vi "Measure_FUN_VISA.vi"(7 "VISA Action":T2, 8 "Error In":errorcluster, 10 "VISA Paremeter":T3={"Baud rate"=19200, "Data bits"=8, "Parity"=enum."None", "Stop bits"=10, "Flow control"=0} {"Flow control" items=["None"=0, "XON/XOFF"=1, "RTS/CTS"=2, "DTR/DSR"=4]; "Stop bits" items=["1.0"=10, "1.5"=15, "2.0"=20]; "Data bits" min=5 max=8 step=1; "Baud rate" items=["75"=75, "110"=110, "134"=134, "150"=150, "300"=300, "600"=600, "1200"=1200, "1800"=1800, "2400"=2400, "4800"=4800, "7200"=7200, "9600"=9600, "14400"=14400, "19200"=19200, "28800"=28800, "38400"=38400, "56000"=56000, "57600"=57600, "115200"=115200, "128000"=128000, "230400"=230400]}, 11 "VISA In":refnum<visa-resource-name>="COM9") -> (0 "Error Out":errorcluster, 2 "State":T1, 3 "VISA Out":refnum<visa-resource-name>="COM9")   [LabVIEW 2015]
uses:
  Control_Measure_VISA action.ctl
  <vilib>/Instr/_visa.llb/VISA Configure Serial Port (Instr).vi
panel:
  in  "Time out":u32=3000
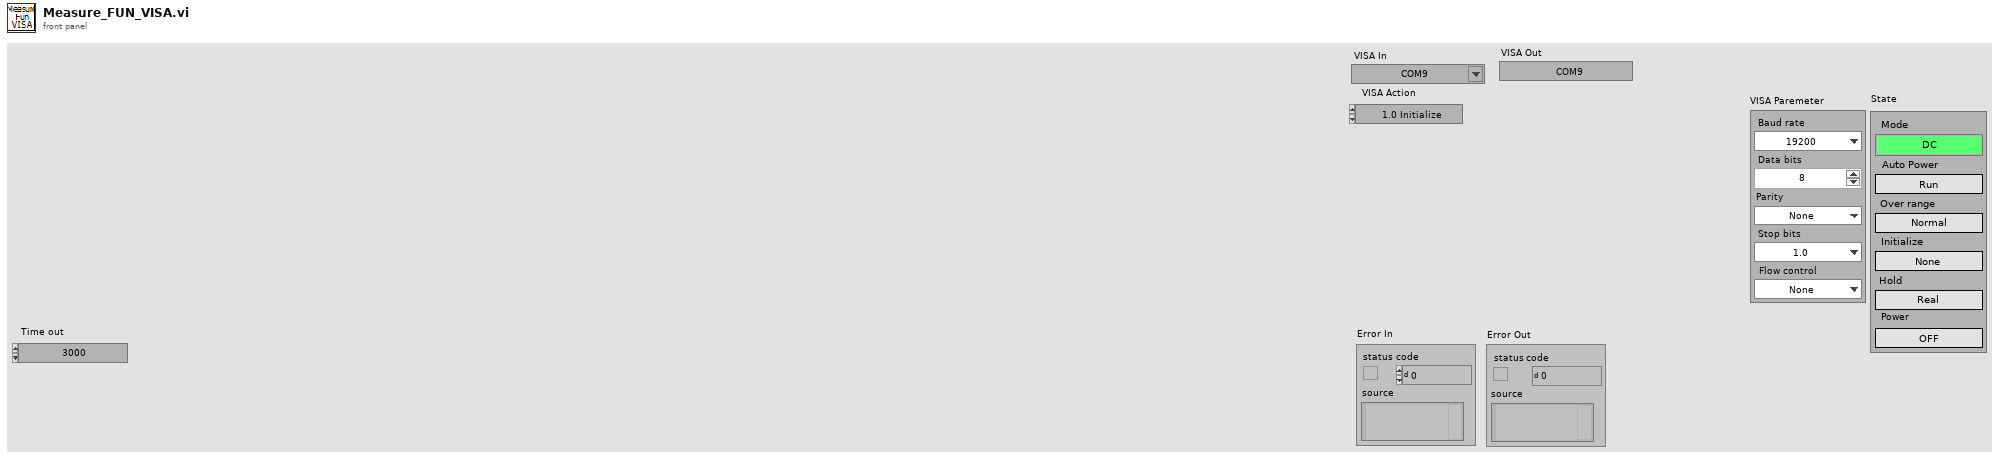
[diagram p1: front panel]
types:
  T1 = cluster{"Mode":enum16{"DC", "DC*10", "AC*10"}, "Auto Power":bool, "Over range":bool, "Initialize":bool, "Hold":bool, "Power":bool}
  T2 = typedef "Control_Measure_VISA action.ctl" = enum16{"1.0 Initialize", "2.0 Power ON", "2.1 Prower OFF", "2.2 Real", "2.3 Hold", "2.4 Reset", "2.5 DC Mode", "2.5.2 DC*10 Mode", "2.5.3 AC*10 Mode", "2.6 Write Commend", "2.7 Write Commend(Power)", "3.0 Read State", "3.1 Read Value", "4.0 Clear", "5.0 Close", "6.0 Idle"}
  T3 = cluster{"Baud rate":u32, "Data bits":u16, "Parity":enum16{"None", "Odd", "Even", "Mark", "Space"}, "Stop bits":u16, "Flow control":u16}
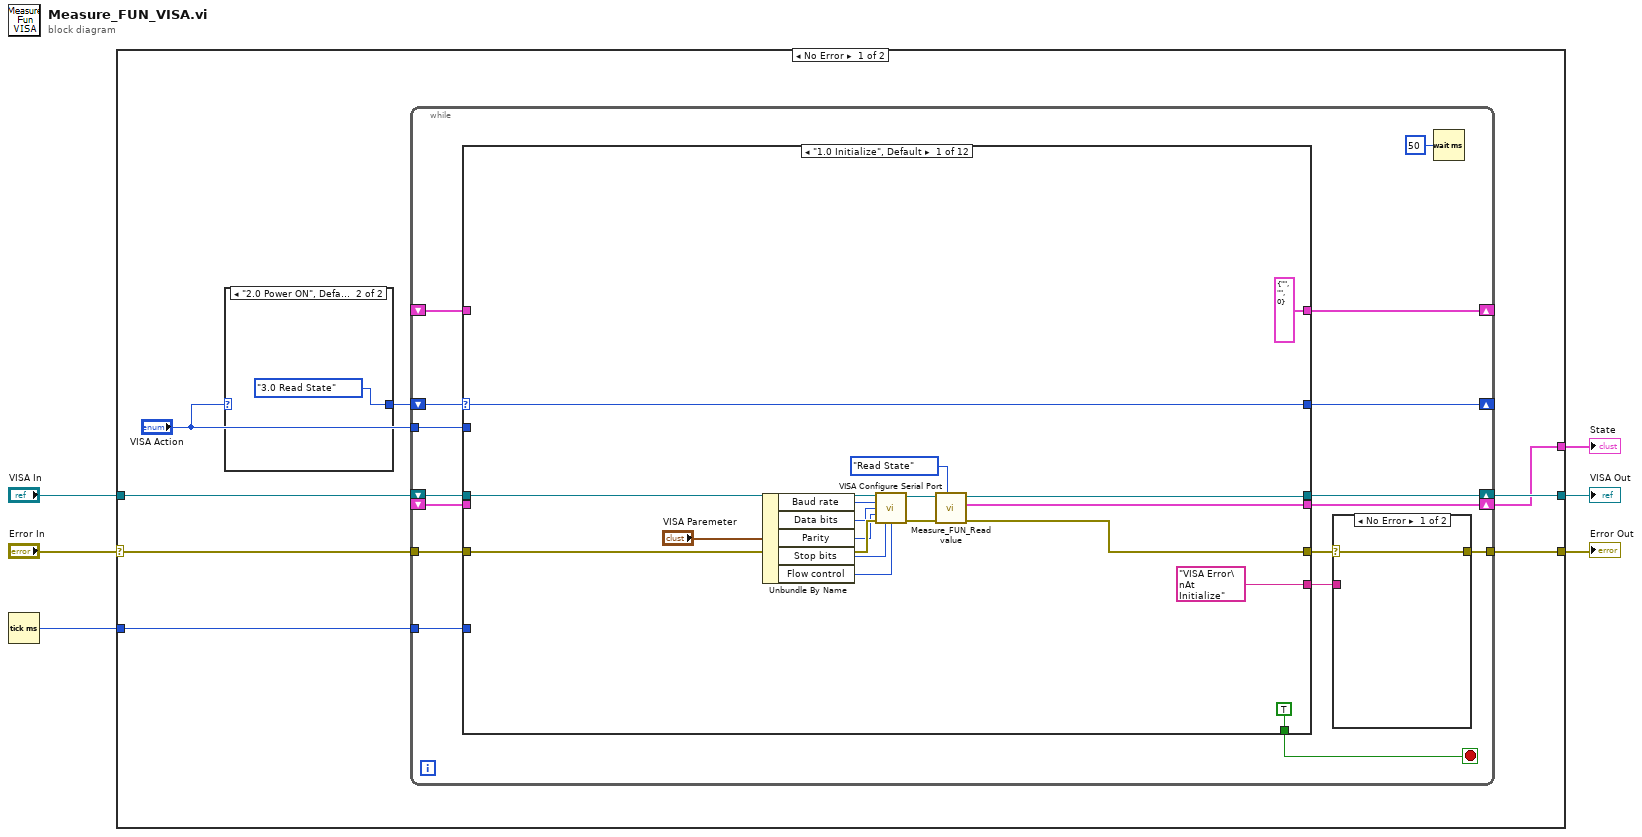
[diagram p0: block diagram]
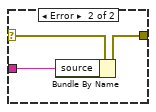
[diagram p3: hidden frame]
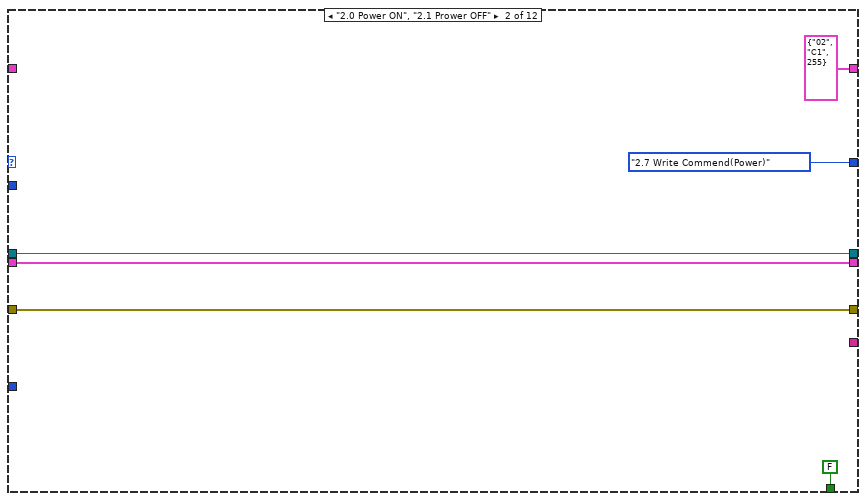
[diagram p4: hidden frame]
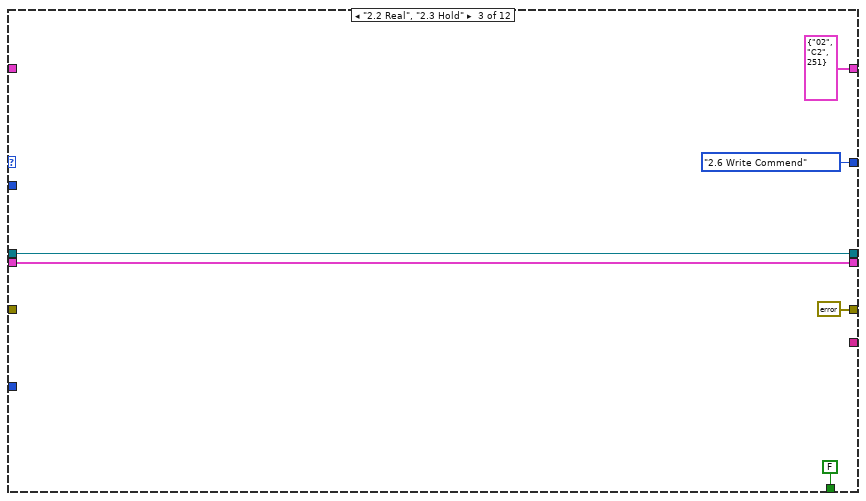
[diagram p5: hidden frame]
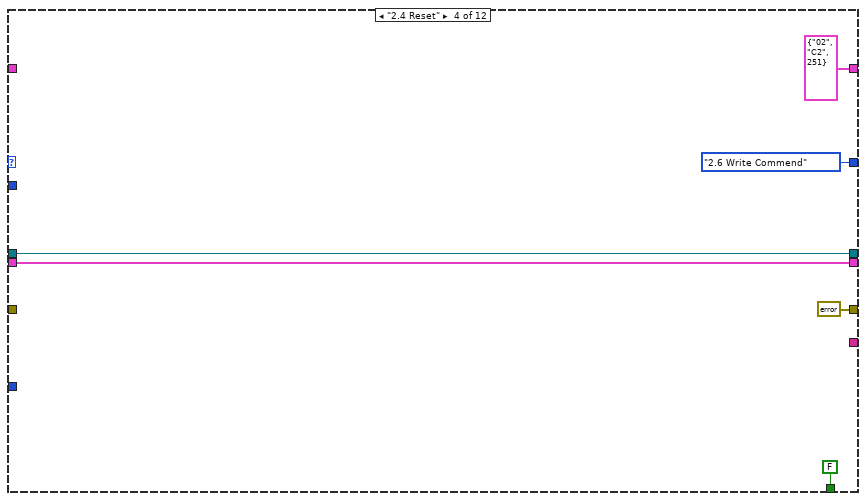
[diagram p6: hidden frame]
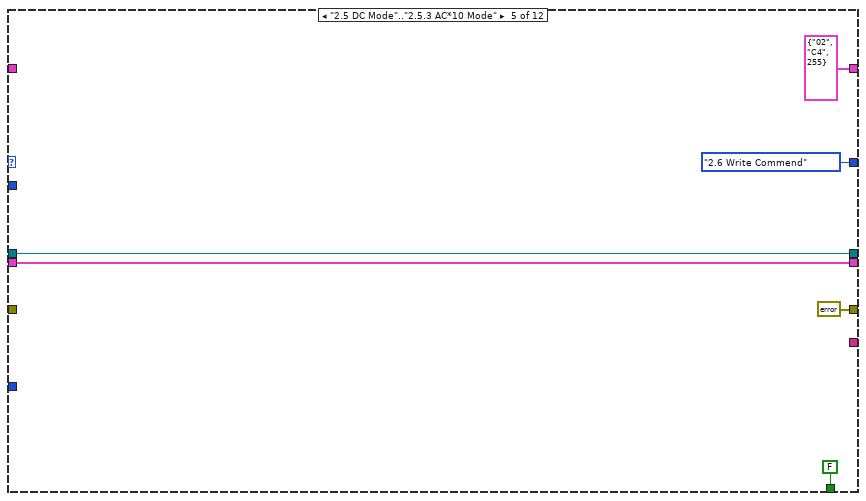
[diagram p7: hidden frame]
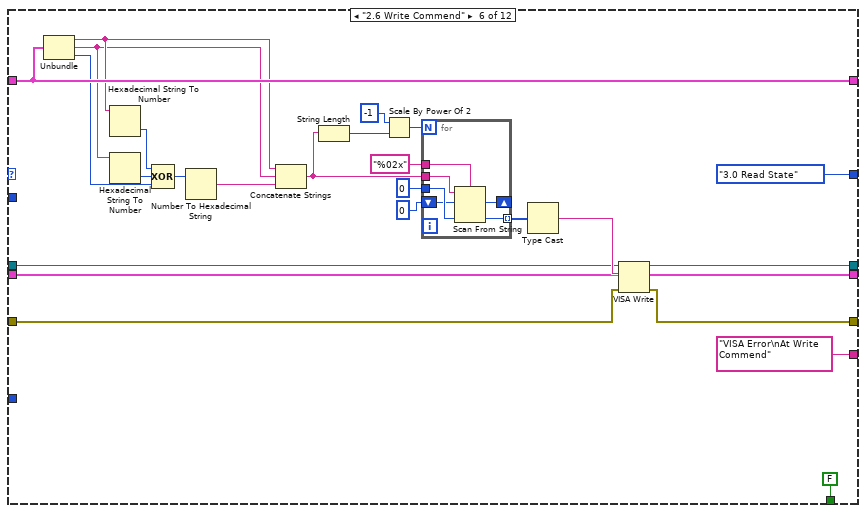
[diagram p8: hidden frame]
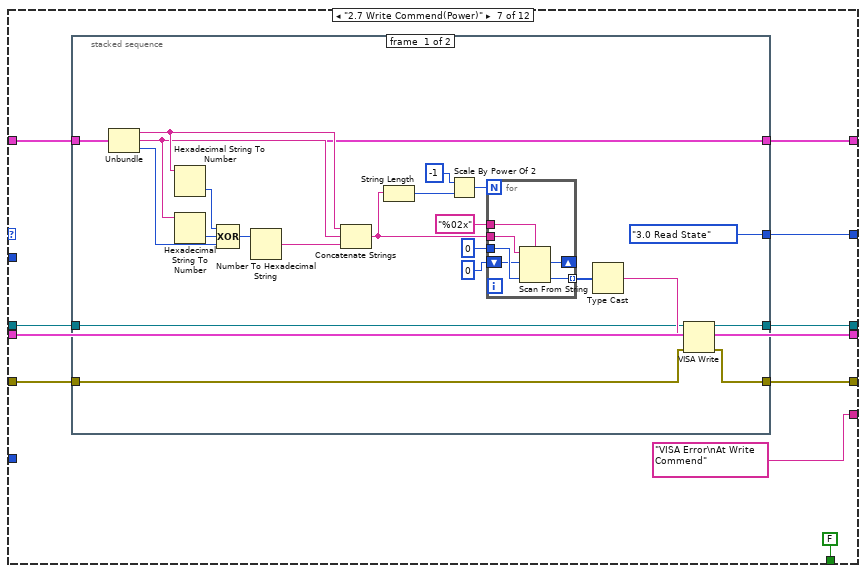
[diagram p9: hidden frame]
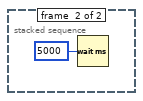
[diagram p10: hidden frame]
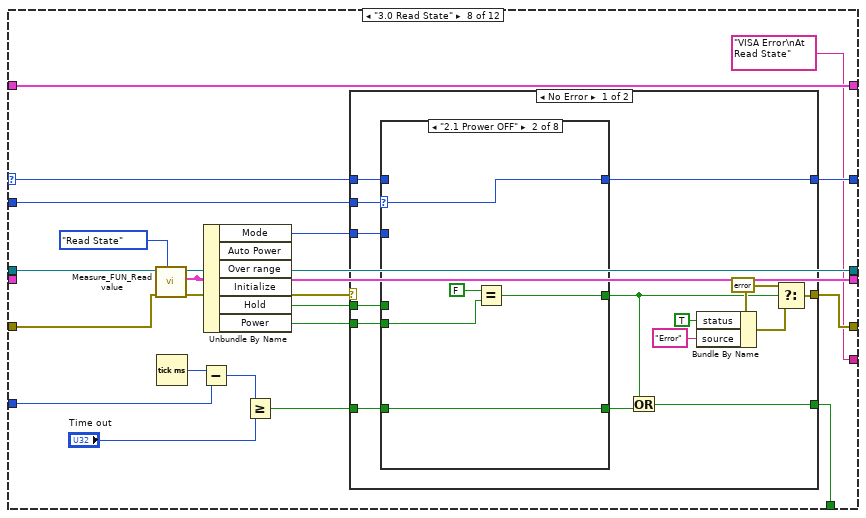
[diagram p11: hidden frame]
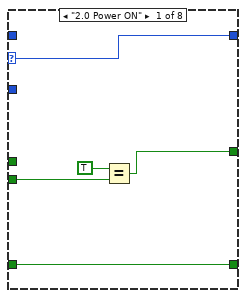
[diagram p12: hidden frame]
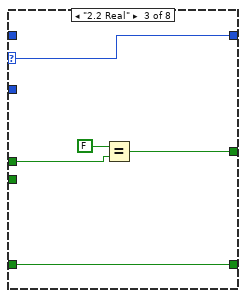
[diagram p13: hidden frame]
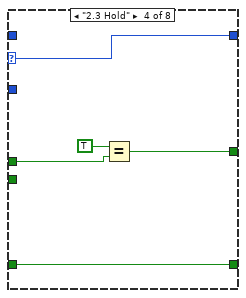
[diagram p14: hidden frame]
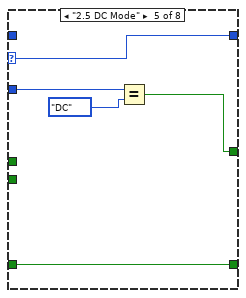
[diagram p15: hidden frame]
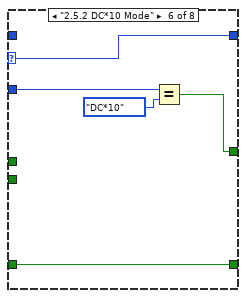
[diagram p16: hidden frame]
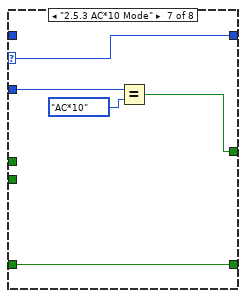
[diagram p17: hidden frame]
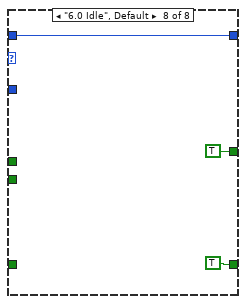
[diagram p18: hidden frame]
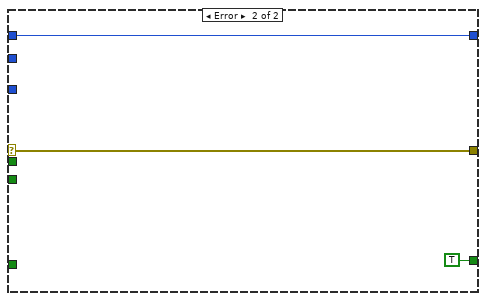
[diagram p19: hidden frame]
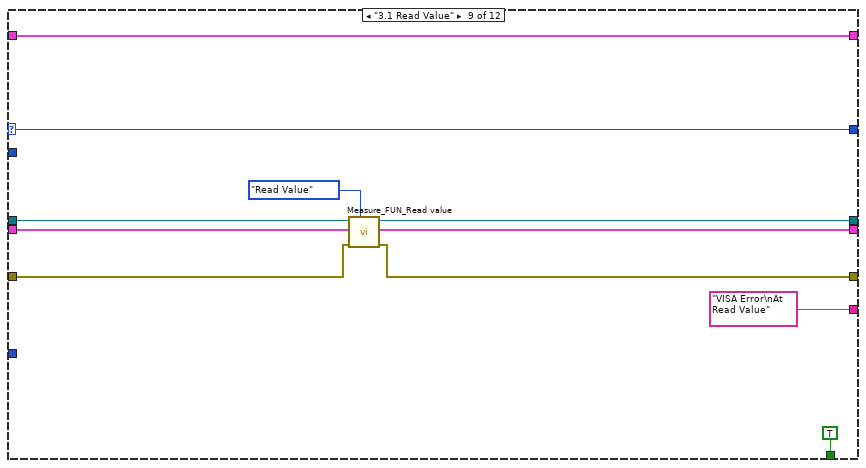
[diagram p20: hidden frame]
diagram:
  n1 = Tick Count (ms)() -> (millisecond timer value=w2:u32)
  n2 = case shown="No Error" "Error In" {
    selector: "Error In" -> [w14 w260]
    tunnel: [w13 w260] -> w5
    tunnel: "VISA In" -> [w12 w259]
    tunnel: [w11 w259] -> w3
    tunnel: w2 -> [w10 _]
    tunnel: [w8 T1 {"Mode"=enum."DC", "Auto Power"=FALSE, "Over range"=FALSE, "Initialize"=FALSE, "Hold"=FALSE, "Power"=FALSE} ("State")] -> w1
    frame No Error {
      n3 = case shown="\"2.0 Power ON\", Default" "VISA Action" {
        selector: "VISA Action" -> [w15 _]
        tunnel: [w15 Control_Measure_VISA_action."3.0 Read State" ("VISA Action")] -> w9
        frame "1.0 Initialize" {
        }
        frame "2.0 Power ON", Default {
        }
      }
      n4 = while {
        shift-right: [w32] -> w11
        shift-left: w12 -> [w31]
        tunnel: w14 -> [w30]
        tunnel: [w18] -> w13
        shift-right: [w29] -> _
        shift-left: _ -> [w28]
        shift-right: [w27] -> _
        shift-left: w9 -> [w25]
        tunnel: w10 -> [w24]
        tunnel: "VISA Action" -> [w23]
        shift-right: [w21] -> w8
        shift-left: _ -> [w20]
        stop <- w26 stop-if-true
        n5 = case shown="\"1.0 Initialize\", Default" w25 {
          selector: w25 -> [w52 _ _ _ _ _ _ w158 w234 w240 w251 w254]
          tunnel: [w46 w60 w66 w70 w76 w102 w119 w167 w231 w243 w248 w256] -> w32
          tunnel: w31 -> [w50 w60 w66 w70 w76 w83 w116 w168 w232 w243 w248 w256]
          tunnel: w30 -> [w54 w59 _ _ _ w82 w117 w166 w230 w242 w247 w255]
          tunnel: [w44 w59 errorcluster {"status"=FALSE, "code"=0, "source"=""} ("error IO") errorcluster {"status"=FALSE, "code"=0, "source"=""} ("error IO") errorcluster {"status"=FALSE, "code"=0, "source"=""} ("error IO") w101 w118 w163 w229 w241 w246 w255] -> w19
          tunnel: [cluster{string, string, u32} {"", "", 0} cluster{string, string, u32} {"02", "C1", 255} cluster{string, string, u32} {"02", "C2", 251} cluster{string, string, u32} {"02", "C2", 251} cluster{string, string, u32} {"02", "C4", 255} w87 w114 w169 w235 w239 w249 w257] -> w29
          tunnel: w28 -> [_ _ _ _ _ w87 w115 w169 w235 w239 w249 w257]
          tunnel: [w52 Control_Measure_VISA_action."2.7 Write Commend(Power)" ("VISA Action") Control_Measure_VISA_action."2.6 Write Commend" ("VISA Action") Control_Measure_VISA_action."2.6 Write Commend" ("VISA Action") Control_Measure_VISA_action."2.6 Write Commend" ("VISA Action") Control_Measure_VISA_action."3.0 Read State" ("VISA Action") w112 w159 w234 w240 w251 w254] -> w27
          tunnel: [TRUE FALSE FALSE FALSE FALSE FALSE FALSE w157 TRUE TRUE TRUE TRUE] -> w26
          tunnel: w23 -> [_ _ _ _ _ _ _ w160 _ _ _ _]
          tunnel: w24 -> [_ _ _ _ _ _ _ w152 _ _ _ _]
          tunnel: [w45 w55 w62 w68 w74 w80 w111 w150 w227 w237 w245 w252] -> w21
          tunnel: w20 -> [_ w55 w62 w68 w74 w80 w111 _ w227 w237 w245 w252]
          tunnel: ["VISA Error\nAt Initialize" _ _ _ _ "VISA Error\nAt Write Commend" "VISA Error\nAt Write Commend" "VISA Error\nAt Read State" "VISA Error\nAt Read Value" "VISA Error\nAt Clear" "VISA Error\nAt Close" _] -> w17
          frame "1.0 Initialize", Default {
            n6 = Unbundle By Name("VISA Paremeter") -> ("Baud rate"=w39:u32, "Data bits"=w40:u16, "Parity"=w41:enum16{"None", "Odd", "Even", "Mark", "Space"}, "Stop bits"=w42:u16, "Flow control"=w43:u16)
            n7 = call-poly "VISA Configure Serial Port"("VISA resource name"=w50, "baud rate (9600)"=w39, "data bits (8)"=w40, "parity (0:none)"=w41, "error in (no error)"=w54, "stop bits (10: 1 bit)"=w42, "flow control (0:none)"=w43) -> ("VISA resource name out"=w48:refnum<visa-resource-name>, "error out"=w47:errorcluster)  [unwired: 2 in, 5 out]
            n8 = call "Measure_FUN_Read value.vi"("Read Action"=enum16{"Initialize", "Read Value", "Read State"}."Read State", "Error In"=w47, "VISA In"=w48) -> ("Error Out"=w44:errorcluster, "State"=w45:T1, "VISA Out"=w46:refnum<visa-resource-name>)  [unwired: 5 in, 1 out]
          }
          frame "2.0 Power ON", "2.1 Prower OFF" {
          }
          frame "2.2 Real", "2.3 Hold" {
          }
          frame "2.4 Reset" {
          }
          frame "2.5 DC Mode".."2.5.3 AC*10 Mode" {
          }
          frame "2.6 Write Commend" {
            n9 = Unbundle(w87) -> (w85:string, w84:string, w81:u32)
            n10 = Hexadecimal String To Number(string=w85) -> (number=w89:u32)  [unwired: 2 in, 1 out]
            n11 = Hexadecimal String To Number(string=w84) -> (number=w90:u32)  [unwired: 2 in, 1 out]
            n12 = Compound Arithmetic op=XOR(w89, w90, w81) -> (w91:u32)
            n13 = Number To Hexadecimal String(2:w91) -> (0:w92:string)  [unwired: 1 in]
            n14 = Concatenate Strings(w85, w84, w92) -> (w88:string)
            n15 = String Length(string=w88) -> (length=w93:i32)
            n16 = Scale By Power Of 2(n=i16 -1, x=w93) -> (x*2^n=w96:i32)
            n17 = for {
              N: w96 -> [_]
              tunnel: w88 -> [w109]
              shift-right: [w105] -> _
              shift-left: u32 0 -> [w106]
              tunnel: "%02x" -> [w107]
              tunnel: [w104] -> w99 mode=indexing
              tunnel: u8 0 -> [w108]
              n18 = Scan From String(format string=w107, input string=w109, initial scan location=w106, default 1=w108) -> (offset past scan=w105:u32, output 1=w104:u8)  [unwired: 1 in, 2 out]
            }
            n19 = Type Cast(x=w99) -> (*(type *) &x=w86:string)  [unwired: 1 in]
            n20 = VISA Write(VISA resource name=w83, write buffer=w86, error in (no error)=w82) -> (VISA resource name out=w102:refnum<visa-resource-name>, error out=w101:errorcluster)  [unwired: 1 out]
          }
          frame "2.7 Write Commend(Power)" {
            n21 = stacked-sequence {
              tunnel: [w125 _] -> w119
              tunnel: [w124 _] -> w118
              tunnel: w117 -> [w123 _]
              tunnel: w116 -> [w122 _]
              tunnel: w115 -> [w121 _]
              tunnel: [w121 _] -> w114
              tunnel: [Control_Measure_VISA_action."3.0 Read State" ("VISA Action") _] -> w112
              frame #0 {
                n22 = Unbundle(w121) -> (w128:string, w127:string, w126:u32)
                n23 = Hexadecimal String To Number(string=w128) -> (number=w131:u32)  [unwired: 2 in, 1 out]
                n24 = Hexadecimal String To Number(string=w127) -> (number=w132:u32)  [unwired: 2 in, 1 out]
                n25 = Compound Arithmetic op=XOR(w131, w132, w126) -> (w133:u32)
                n26 = Number To Hexadecimal String(2:w133) -> (0:w134:string)  [unwired: 1 in]
                n27 = Concatenate Strings(w128, w127, w134) -> (w130:string)
                n28 = String Length(string=w130) -> (length=w135:i32)
                n29 = Scale By Power Of 2(n=i16 -1, x=w135) -> (x*2^n=w138:i32)
                n30 = for {
                  N: w138 -> [_]
                  tunnel: w130 -> [w147]
                  shift-right: [w143] -> _
                  shift-left: u32 0 -> [w144]
                  tunnel: "%02x" -> [w145]
                  tunnel: [w142] -> w141 mode=indexing
                  tunnel: u8 0 -> [w146]
                  n31 = Scan From String(format string=w145, input string=w147, initial scan location=w144, default 1=w146) -> (offset past scan=w143:u32, output 1=w142:u8)  [unwired: 1 in, 2 out]
                }
                n32 = Type Cast(x=w141) -> (*(type *) &x=w129:string)  [unwired: 1 in]
                n33 = VISA Write(VISA resource name=w122, write buffer=w129, error in (no error)=w123) -> (VISA resource name out=w125:refnum<visa-resource-name>, error out=w124:errorcluster)  [unwired: 1 out]
              }
              frame #1 {
                n34 = Wait (ms)(milliseconds to wait=u32 5000) -> ()  [unwired: 1 out]
              }
            }
          }
          frame "3.0 Read State" {
            n35 = call "Measure_FUN_Read value.vi"("Read Action"=enum16{"Initialize", "Read Value", "Read State"}."Read State", "Error In"=w166, "VISA In"=w168) -> ("Error Out"=w164:errorcluster, "State"=w150:T1, "VISA Out"=w167:refnum<visa-resource-name>)  [unwired: 5 in, 1 out]
            n36 = Tick Count (ms)() -> (millisecond timer value=w154:u32)
            n37 = Subtract(x=w154, y=w152) -> (x-y=w155:u32)
            n38 = Unbundle By Name(w150) -> ("Mode"=w161:enum16{"DC", "DC*10", "AC*10"}, "Hold"=w162:bool, "Power"=w165:bool)  [unwired: 3 out]
            n39 = Greater Or Equal?(x=w155, y="Time out") -> (x >= y?=w153:bool)
            n40 = case shown="No Error" w164 {
              selector: w164 -> [_ w225]
              tunnel: w165 -> [w178 _]
              tunnel: [w184 w225] -> w163
              tunnel: w162 -> [w177 _]
              tunnel: w161 -> [w176 _]
              tunnel: w160 -> [w179 _]
              tunnel: [w175 w224] -> w159
              tunnel: w158 -> [w174 w224]
              tunnel: [w171 TRUE] -> w157
              tunnel: w153 -> [w173 _]
              frame No Error {
                w182 = errorcluster {"status"=FALSE, "code"=0, "source"=""} ("Error Out")
                n41 = case shown="\"2.1 Prower OFF\"" w179 {
                  selector: w179 -> [w186 w191 w196 w201 w206 w211 w216 _]
                  tunnel: w178 -> [w189 w192 _ _ _ _ _ _]
                  tunnel: [w188 w193 w198 w203 w207 w212 w217 TRUE] -> w170
                  tunnel: w177 -> [_ _ w197 w202 _ _ _ _]
                  tunnel: w176 -> [_ _ _ _ w208 w214 w218 _]
                  tunnel: [w186 w191 w196 w201 w206 w211 w216 w221] -> w175
                  tunnel: w174 -> [_ _ _ _ _ _ _ w221]
                  tunnel: [w185 w190 w195 w200 w205 w210 w215 TRUE] -> w172
                  tunnel: w173 -> [w185 w190 w195 w200 w205 w210 w215 _]
                  frame "2.0 Power ON" {
                    n42 = Equal?(x=TRUE, y=w189) -> (x = y?=w188:bool)
                  }
                  frame "2.1 Prower OFF" {
                    n43 = Equal?(x=FALSE, y=w192) -> (x = y?=w193:bool)
                  }
                  frame "2.2 Real" {
                    n44 = Equal?(x=FALSE, y=w197) -> (x = y?=w198:bool)
                  }
                  frame "2.3 Hold" {
                    n45 = Equal?(x=TRUE, y=w202) -> (x = y?=w203:bool)
                  }
                  frame "2.5 DC Mode" {
                    n46 = Equal?(x=w208, y=enum16{"DC", "DC*10", "AC*10"}."DC" ("Mode")) -> (x = y?=w207:bool)
                  }
                  frame "2.5.2 DC*10 Mode" {
                    n47 = Equal?(x=w214, y=enum16{"DC", "DC*10", "AC*10"}."DC*10" ("Mode")) -> (x = y?=w212:bool)
                  }
                  frame "2.5.3 AC*10 Mode" {
                    n48 = Equal?(x=w218, y=enum16{"DC", "DC*10", "AC*10"}."AC*10" ("Mode")) -> (x = y?=w217:bool)
                  }
                  frame "6.0 Idle", Default {
                  }
                }
                n49 = Or(x=w170, y=w172) -> (x .or. y?=w171:bool)
                n50 = Bundle By Name(cluster=w182, "status"=TRUE, "source"="Error") -> (w183:errorcluster)
                n51 = Select(t=w182, s=w170, f=w183) -> (s? t:f=w184:errorcluster)
              }
              frame Error {
              }
            }
          }
          frame "3.1 Read Value" {
            n52 = call "Measure_FUN_Read value.vi"("Read Action"=enum16{"Initialize", "Read Value", "Read State"}."Read Value", "Error In"=w230, "VISA In"=w232) -> ("Error Out"=w229:errorcluster, "VISA Out"=w231:refnum<visa-resource-name>)  [unwired: 5 in, 2 out]
          }
          frame "4.0 Clear" {
            n53 = VISA Clear(VISA resource name=w243, error in (no error)=w242) -> (error out=w241:errorcluster)  [unwired: 1 out]
          }
          frame "5.0 Close" {
            n54 = VISA Close(VISA resource name=w248, error in (no error)=w247) -> (error out=w246:errorcluster)
          }
          frame "6.0 Idle" {
          }
        }
        n55 = case shown="No Error" w19 {
          selector: w19 -> [w33 w36]
          tunnel: [w33 w35] -> w18
          tunnel: w17 -> [_ w34]
          frame No Error {
          }
          frame Error {
            n56 = Bundle By Name(cluster=w36, "source"=w34) -> (w35:errorcluster)
          }
        }
        n57 = Wait (ms)(milliseconds to wait=u32 50) -> ()  [unwired: 1 out]
      }
    }
    frame Error {
    }
  }
  "Error Out" <- w5
  "VISA Out" <- w3
  "State" <- w1
